vi "Get Font Size.vi"(7 "Height":u32) -> (8 "Font Size":i32)   [LabVIEW 2011]
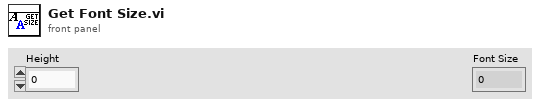
[diagram p1: front panel]
types:
  T1 = cluster{"Font Name:":string, "Size":i16, "Strikeout?":bool, "Italic?":bool, "Underline?":bool, "Outline?":bool, "Shadow?":bool, "Bold?":bool}
  T2 = enum16{"User-specified Font", "Application Font", "System Font", "Dialog Font"}
  T3 = cluster{"left":i16, "top":i16, "right":i16, "bottom":i16}
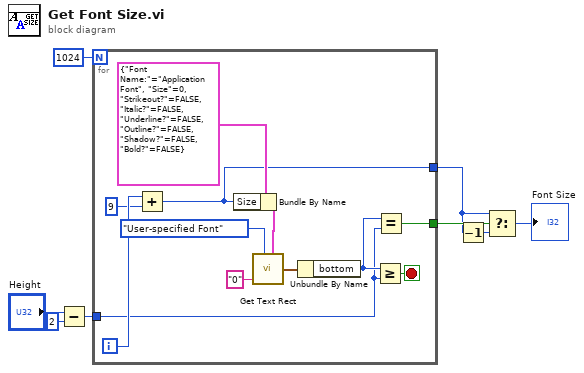
[diagram p0: block diagram]
diagram:
  n1 = Subtract(x="Height", y=u32 2) -> (x-y=w2:u32)
  n2 = for {
    N: 1024 -> [_]
    tunnel: w2 -> [w10]
    tunnel: [w13] -> w6
    tunnel: [w9] -> w7
    i -> [w14]
    stop <- w15 stop-if-true
    n3 = Add(x=w14, y=9) -> (x+y=w13:i32)
    n4 = Bundle By Name(cluster=T1 {"Font Name:"="Application Font", "Size"=0, "Strikeout?"=FALSE, "Italic?"=FALSE, "Underline?"=FALSE, "Outline?"=FALSE, "Shadow?"=FALSE, "Bold?"=FALSE} ("[user-specified font]"), "Size"=w13) -> (w16:T1)
    n5 = call <vilib>:"Get Text Rect.vi"("desired font(Application)"=T2."User-specified Font", "text"="0", "[user-specified font]"=w16) -> ("rect"=w19:T3)  [unwired: 6 in]
    n6 = Unbundle By Name(w19) -> ("bottom"=w11:i16)
    n7 = Greater Or Equal?(x=w11, y=w10) -> (x >= y?=w15:bool)
    n8 = Equal?(x=w11, y=w10) -> (x = y?=w9:bool)
  }
  n9 = Decrement(x=w6) -> (x-1=w5:i32)
  n10 = Select(t=w6, s=w7, f=w5) -> (s? t:f=→"Font Size":i32)
